vi "Generate Start-Up Registry Patch File.vi"(6 "registry path":T1(ring), 7 "Registry File Path":path, 8 "error in (no error)":errorcluster, 9 "Key Name(Empty to use exe name)":string, 10 "Arguments":string, 11 "EXE Path":path) -> (0 "error out":errorcluster)   [LabVIEW 2017]
doc: "Writes a .reg patch file that adds EXE Path to one of the Windows run or run-once registry keys, so the application starts automatically. Key Name defaults to the executable name, and Arguments is appended to the command line."
uses:
  kernel32.dll
  Configuration/Ini/ini_configuration.lvlib
panel:
  out "resulting string":string
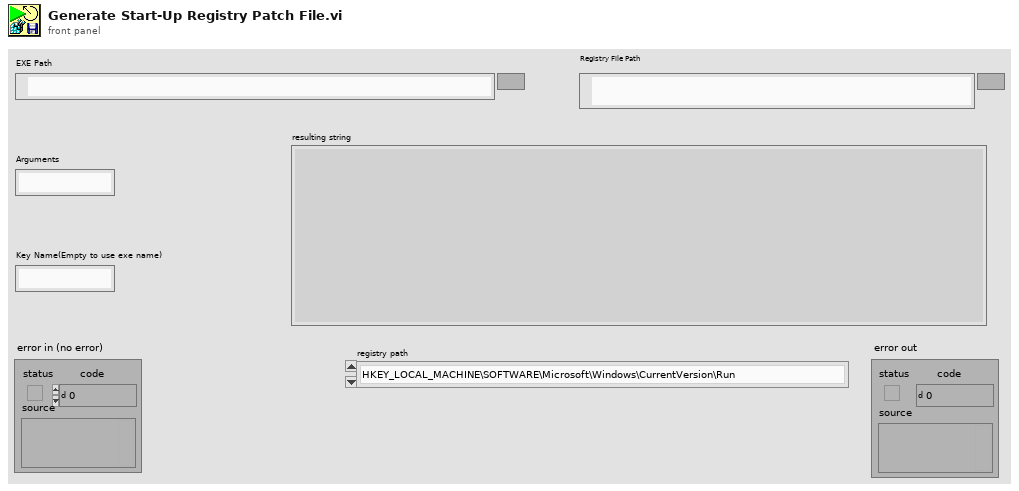
[diagram p1: front panel]
types:
  T1 = enum16{"HKEY_LOCAL_MACHINE\\SOFTWARE\\Microsoft\\Windows\\CurrentVersion\\Run", "HKEY_LOCAL_MACHINE\\Software\\Microsoft\\Windows\\CurrentVersion\\RunOnce", "HKEY_CURRENT_USER\\Software\\Microsoft\\Windows\\CurrentVersion\\Run", "HKEY_CURRENT_USER\\Software\\Microsoft\\Windows\\CurrentVersion\\RunOnce"}
  T2 = enum16{"open", "replace", "create", "open or create", "replace or create", "replace or create with confirmation"}
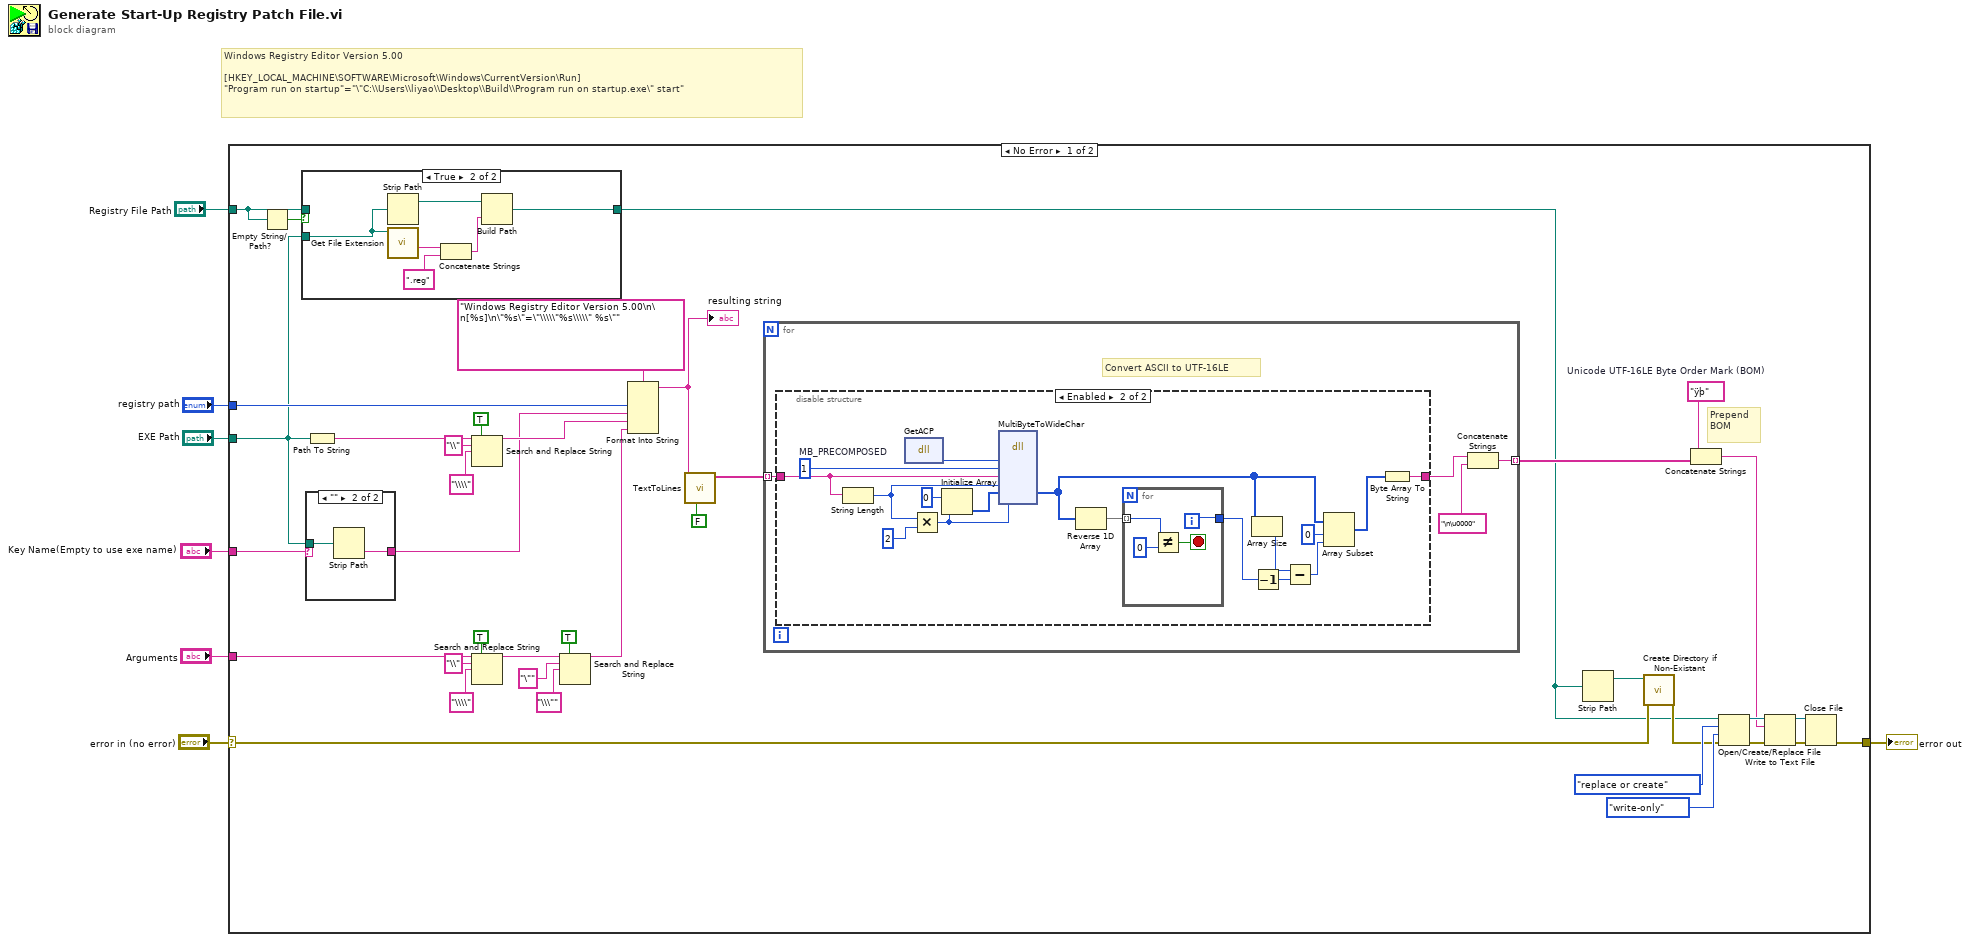
[diagram p0: block diagram]
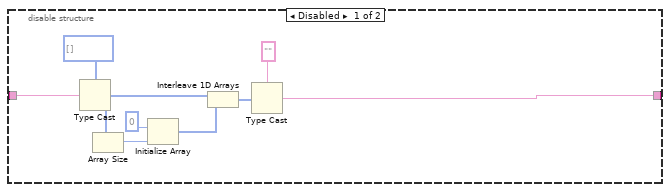
[diagram p3: hidden frame]
diagram:
  # "Windows Registry Editor Version 5.00\n\n[HKEY_LOCAL_MACHINE\\SOFTWARE\\Microsoft\\Windows\\CurrentVersion\\Run]\n\"Program run on startup\"=\"\\\"C:\\\\Users\\\\liyao\\\\Desktop\\\\Build\\\\Program run on startup.exe\\\" start\""
  n1 = case shown="No Error" "error in (no error)" {
    selector: "error in (no error)" -> [w18 w90]
    tunnel: "registry path" -> [w45 _]
    tunnel: "EXE Path" -> [w10 _]
    tunnel: "Key Name(Empty to use exe name)" -> [w40 _]
    tunnel: "Arguments" -> [w36 _]
    tunnel: [w17 w90] -> w2
    tunnel: "Registry File Path" -> [w9 _]
    frame No Error {
      w16 = "ÿþ"  # Unicode UTF-16LE Byte Order Mark (BOM)
      # "Prepend\nBOM"
      n2 = Empty String/Path?(string/path=w9) -> (empty?=w11:bool)
      n3 = case shown="True" w11 {
        tunnel: w9 -> [w46 _]
        tunnel: [w46 w47] -> w8
        tunnel: w10 -> [_ w48]
        frame False {
        }
        frame True {
          n4 = Strip Path(path=w48) -> (stripped path=w52:path)  [unwired: 1 out]
          n5 = call <vilib>:"Get File Extension.vi"("file"=w48) -> ("filename without extension"=w51:string)  [unwired: 6 in, 4 out]
          n6 = Concatenate Strings(w51, ".reg" ("string")) -> (w50:string)
          n7 = Build Path(base path=w52, name or relative path=w50) -> (appended path=w47:path)
        }
      }
      n8 = case shown="\"\"" w40 {
        selector: w40 -> [w87 _]
        tunnel: w10 -> [_ w89]
        tunnel: [w87 w88] -> w28
        frame "False", Default {
        }
        frame "" {
          n9 = Strip Path(path=w89) -> (name=w88:string)  [unwired: 1 out]
        }
      }
      n10 = Path To String(path=w10) -> (string=w44:string)
      n11 = Search and Replace String(replace all?=TRUE ("replace all? (F)"), input string=w44, search string="\\", replace string="\\\\" ("search string")) -> (result string=w29:string)  [unwired: 4 in, 3 out]
      n12 = Search and Replace String(replace all?=TRUE ("replace all? (F)"), input string=w36, search string="\\", replace string="\\\\" ("search string")) -> (result string=w32:string)  [unwired: 4 in, 3 out]
      n13 = Search and Replace String(replace all?=TRUE ("replace all? (F)"), input string=w32, search string="\"", replace string="\\\"" ("search string")) -> (result string=w30:string)  [unwired: 4 in, 3 out]
      n14 = Format Into String(format string="Windows Registry Editor Version 5.00\n\n[%s]\n\"%s\"=\"\\\\\"%s\\\\\" %s\"", w45, w28, w29, w30) -> (resulting string=w27:string)  [unwired: 2 in, 1 out]
      "resulting string" <- w27
      n15 = call "TextToLines.vi"("Remove Empty Lines?(T)"=FALSE, "string"=w27) -> ("Lines"=w13:string[])  [unwired: 8 in, 1 out]
      n16 = for {
        tunnel: w13 -> [w56] mode=indexing
        tunnel: [w54] -> w12 mode=indexing
        # "Convert ASCII to UTF-16LE"
        n17 = disable-structure shown="Enabled" {
          disable-tunnel: w56 -> [w65 w76]
          disable-tunnel: [w57 w75] -> w55
          frame Disabled {
            n18 = Type Cast(type=u8[] [], x=w65) -> (*(type *) &x=w61:u8[])
            n19 = Array Size(array=w61) -> (size(s)=w63:i32)
            n20 = Initialize Array(u8 0, w63) -> (w60:u8[])
            n21 = Interleave 1D Arrays(w61, w60) -> (w59:u8[])
            n22 = Type Cast(type="", x=w59) -> (*(type *) &x=w57:string)
          }
          frame Enabled {
            w81 = u32 1  # MB_PRECOMPOSED
            n23 = String Length(string=w76) -> (length=w74:i32)
            n24 = dll-call lib="kernel32.dll" fn="GetACP" label="GetACP()"() -> (w77:u32)  [unwired: 3 in, 2 out]
            n25 = Multiply(x=w74, y=2) -> (x*y=w78:i32)
            n26 = Initialize Array(u8 0, w78) -> (w79:u8[])
            n27 = dll-call lib="kernel32.dll" fn="MultiByteToWideChar"("codePage"=w77, "dwFlags"=w81, "pMultiByteStr"=w76, "cbMultiByte"=w74, "lpWideCharStr"=w79, "cchWideChar"=w78) -> ("lpWideCharStr"=w68:u8[])  [unwired: 8 in, 3 out]
            n28 = Reverse 1D Array(array=w68) -> (reversed array=w73:u8[])
            n29 = for {
              tunnel: w73 -> [w84] mode=indexing
              tunnel: [w83] -> w71
              i -> [w83]
              stop <- w85 stop-if-true
              n30 = Not Equal?(x=w84, y=u8 0) -> (x != y?=w85:bool)
            }
            n31 = Array Size(array=w68) -> (size(s)=w70:i32)
            n32 = Decrement(x=w71) -> (x-1=w66:i32)
            n33 = Subtract(x=w70, y=w66) -> (x-y=w69:i32)
            n34 = Array Subset(array=w68, index=0, length=w69) -> (w67:u8[])
            n35 = Byte Array To String(unsigned byte array=w67) -> (string=w75:string)
          }
        }
        n36 = Concatenate Strings(w55, "\n\u0000" ("delimiter (Tab)")) -> (w54:string)
      }
      n37 = Strip Path(path=w8) -> (stripped path=w20:path)  [unwired: 1 out]
      n38 = call "Create Directory if Non-Existant.vi"("error in (no error)"=w18, "Directory Path"=w20) -> ("error out"=w19:errorcluster)  [unwired: 7 in, 2 out]
      n39 = Concatenate Strings(w16, w12) -> (w15:string)
      n40 = Open/Create/Replace File(file path (use dialog)=w8, error in=w19, operation (0:open)=T2."replace or create", access (0:read/write)=enum16{"read/write", "read-only", "write-only"}."write-only") -> (refnum out=w24:refnum<file>, error out=w21:errorcluster)  [unwired: 2 in, 1 out]
      n41 = Write to Text File(file (use dialog)=w24, text=w15, error in=w21) -> (refnum out=w23:refnum<file>, error out=w22:errorcluster)  [unwired: 1 in, 1 out]
      n42 = Close File(refnum=w23, error in=w22) -> (error out=w17:errorcluster)  [unwired: 1 out]
    }
    frame Error {
    }
  }
  "error out" <- w2
